vi "Add Channel Node.vi"(7 "Channel UI Controls":T1, 11 "Doc Ref":refnum<k20>) -> (2 "Updated Node Ref":refnum<k20>)   [LabVIEW 2025]
uses:
  Types/New Node Types.ctl
  Types/Channel UI Controls.ctl
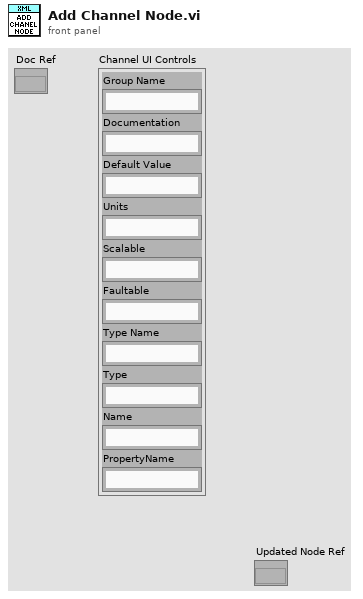
[diagram p1: front panel]
types:
  T1 = typedef "Channel UI Controls.ctl" = cluster{"Group Name":string, "Documentation":string, "Default Value":string, "Units":string, "Scalable":string, "Faultable":string, "Type Name":string, "Type ":string, "Name":string, "PropertyName":string}
  T2 = typedef "New Node Types.ctl" = enum16{"Channel", "Waveform", "Section"}
  T3 = cluster{"Tag Name":string, "Documentation":string}
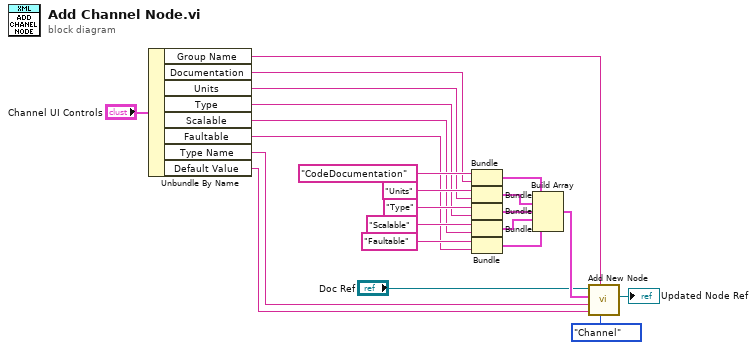
[diagram p0: block diagram]
diagram:
  n1 = Unbundle By Name("Channel UI Controls") -> ("Group Name"=w13:string, "Documentation"=w12:string, "Units"=w11:string, "Type"=w2:string, "Scalable"=w7:string, "Faultable"=w6:string, "Type Name"=w3:string, "Default Value"=w10:string)
  n2 = Bundle("Tag Name"="CodeDocumentation", "Documentation"=w12) -> (w18:T3)  [unwired: 1 in]
  n3 = Bundle("Tag Name"="Units", "Units"=w11) -> (w19:cluster{"Tag Name":string, "Units":string})  [unwired: 1 in]
  n4 = Bundle("Tag Name"="Type", "Type"=w2) -> (w17:cluster{"Tag Name":string, "Type ":string})  [unwired: 1 in]
  n5 = Bundle("Tag Name"="Scalable", "Scalable"=w7) -> (w5:cluster{"Tag Name":string, "Scalable":string})  [unwired: 1 in]
  n6 = Bundle("Tag Name"="Faultable", "Faultable"=w6) -> (w4:cluster{"Tag Name":string, "Faultable":string})  [unwired: 1 in]
  n7 = Build Array(w18, w19, w17, w5, w4) -> (w16:cluster{"Tag Name":string, "Faultable":string}[])
  n8 = call "Add New Node.vi"("New Node Types"=New_Node_Types."Channel", "Group Name"=w13, "Default Element Value"=w10, "Type Name"=w3, "Text Nodes"=w16, "Doc Ref"="Doc Ref") -> ("Updated Node Ref"=→"Updated Node Ref":refnum<k20>)  [unwired: 5 in]
